vi "Write Force Sensor Channel.vi"(8 "error in (no error)":errorcluster, 10 "fs phys chan":tag, 11 "DAQmx Force Sensor in":refnum<class "DAQmx Force Sensor.lvclass">) -> (0 "error out":errorcluster, 3 "DAQmx Force Sensor out":refnum<class "DAQmx Force Sensor.lvclass">)   [LabVIEW 2020, in "DAQmx Force Sensor.lvclass"]
uses:
  DAQmx Force Sensor.lvclass
  DAQmx Force Sensor.lvclass/DAQmx Force Sensor.ctl
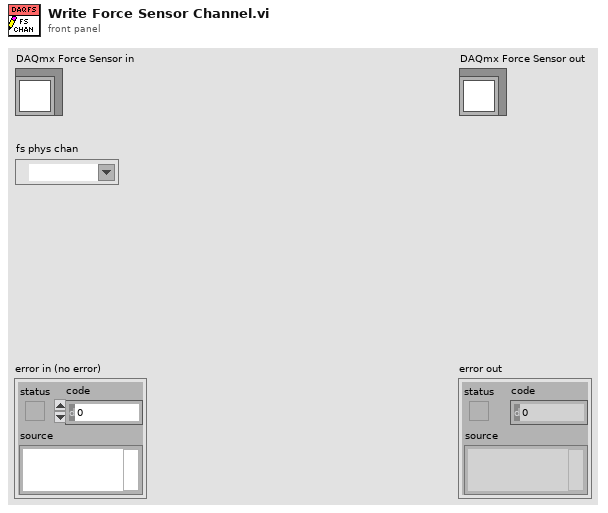
[diagram p1: front panel]
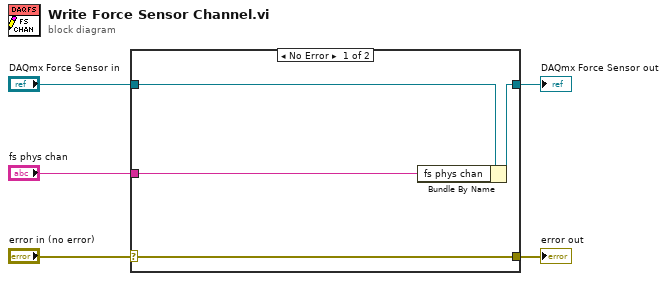
[diagram p0: block diagram]
diagram:
  n1 = case shown="No Error" "error in (no error)" {
    selector: "error in (no error)" -> [w9 w10]
    tunnel: [w9 w10] -> w4
    tunnel: [w7 w11] -> w2
    tunnel: "DAQmx Force Sensor in" -> [w8 w11]
    tunnel: "fs phys chan" -> [w6 _]
    frame No Error {
      n2 = Bundle By Name(cluster=w8, "fs phys chan"=w6) -> (w7:refnum<class "DAQmx Force Sensor.lvclass">)
    }
    frame Error {
    }
  }
  "error out" <- w4
  "DAQmx Force Sensor out" <- w2
